vi "WSVCAP SHL Host LL I2C Write.vi"(0 "C1 Data Out [DUT Ordered]":u8[][](array[numeric]) format="%.0x", 1 "Wait Ticks":u32, 2 "Slave Address":u8, 5 "C2 Data Out [DUT Ordered]":u8[][](array[numeric]) format="%.0x", 7 "C3 Data Out [DUT Ordered]":u8[][](array[numeric]) format="%.0x", 9 "Socket Mask [U64]":u64=1 format="%016x", 11 "error in":errorcluster, 12 "Sub Address":u8=20, 13 "UUT Set (0/1)":u8) -> (10 "Status":u8[](array[numeric]), 15 "error out":errorcluster)   [LabVIEW 2012]
uses:
  Type Defs/WSVCAP SHL Top Level Write Read State Enum.ctl
  Type Defs/WSVCAP SHL Transaction Enum.ctl
  Type Defs/WSVCAP SHL Top Level Control Enum.ctl
  Type Defs/WSVCAP SHL State.ctl
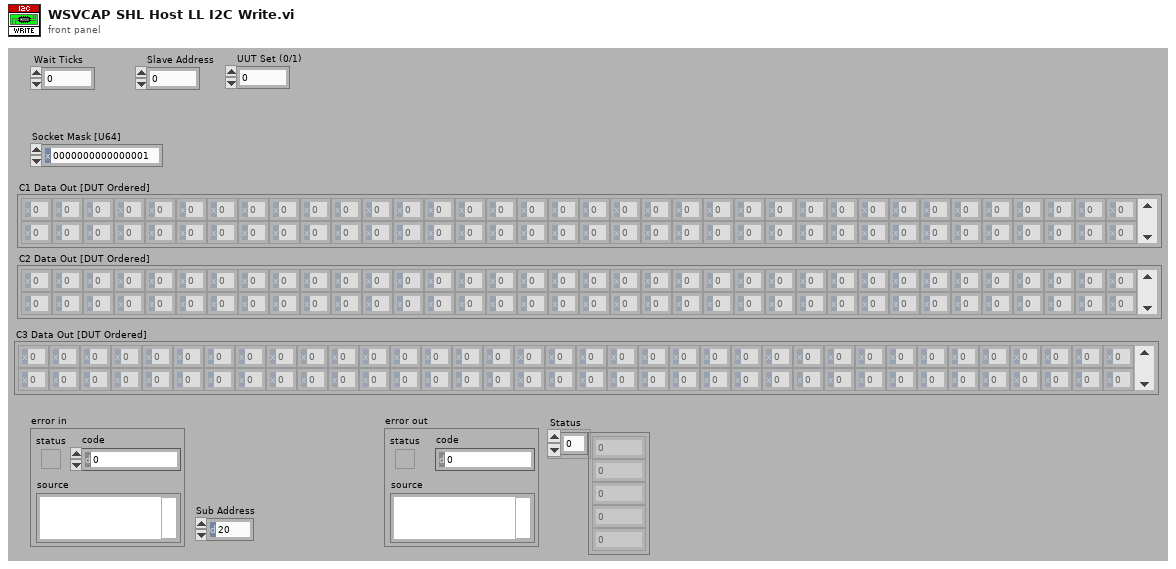
[diagram p1: front panel]
types:
  T1 = typedef "WSVCAP SHL Top Level Write Read State Enum.ctl" = enum16{"Start", "Write", "Read", "Get Status", "Wait Until Done"}
  T2 = typedef "WSVCAP SHL Top Level Control Enum.ctl" = enum16{"Start", "Cmd", "Transaction", "Wait Ticks", "Socket Mask", "UUT Set", "Slave Address", "Sub Address", "Bytes to Write", "Bytes to Read", "Write Data", "Write Flag", "Read Data", "Read Flag", "Ack Read", "Read Status Flag", "Ack Read Status", "Status", "Cycle Count", "Stop Cycle", "Exit"}
  T3 = typedef "WSVCAP SHL Transaction Enum.ctl" = enum16{"I2C-Read Data", "I2C-Write Data", "RFFE-Ext Write", "RFFE-Ext Read"}
  T4 = typedef "WSVCAP SHL State.ctl" = enum8{"Idle", "Transfer Data"}
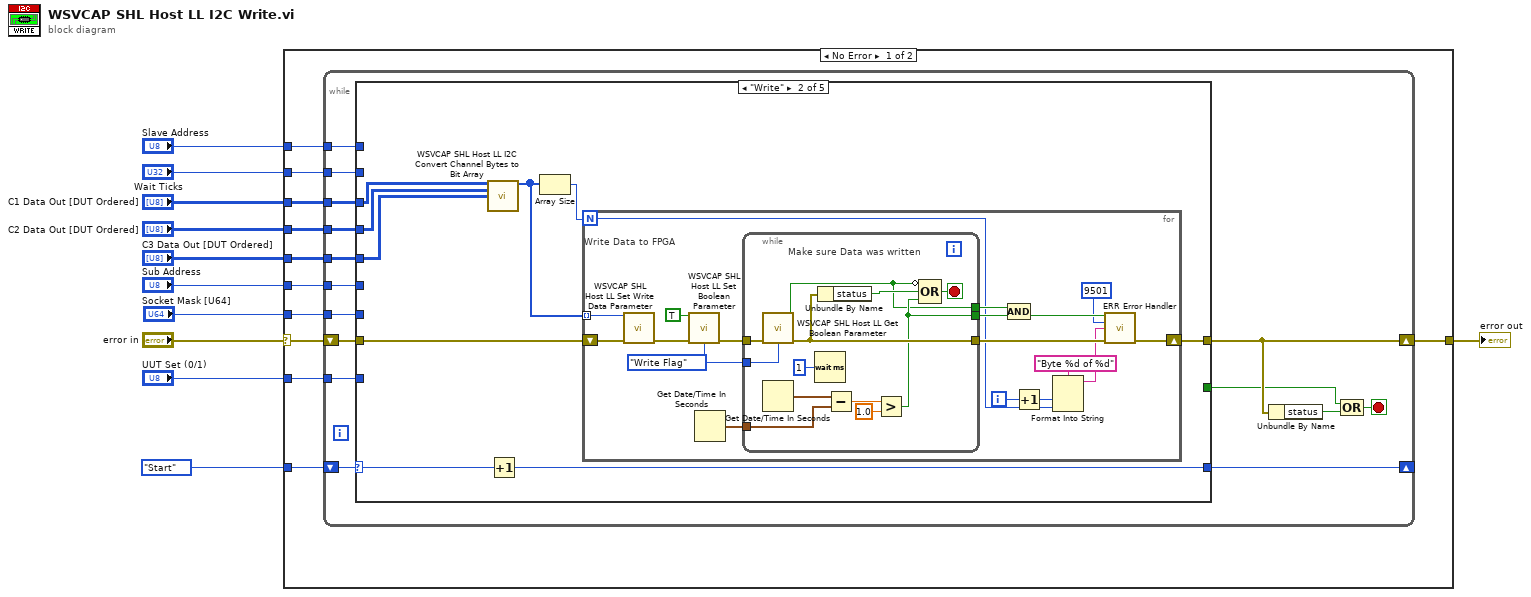
[diagram p0: block diagram]
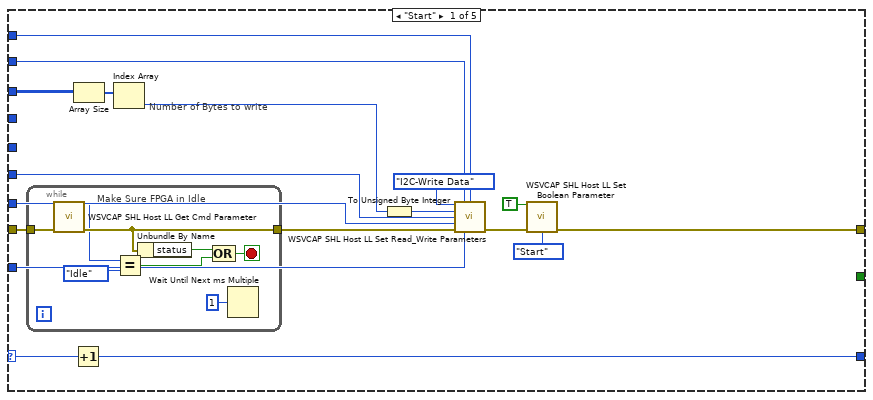
[diagram p2: hidden frame]
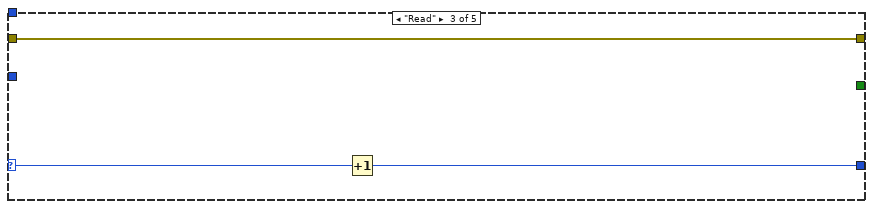
[diagram p3: hidden frame]
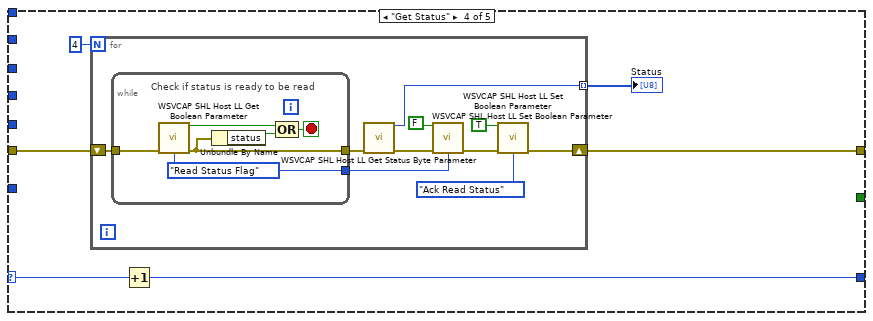
[diagram p4: hidden frame]
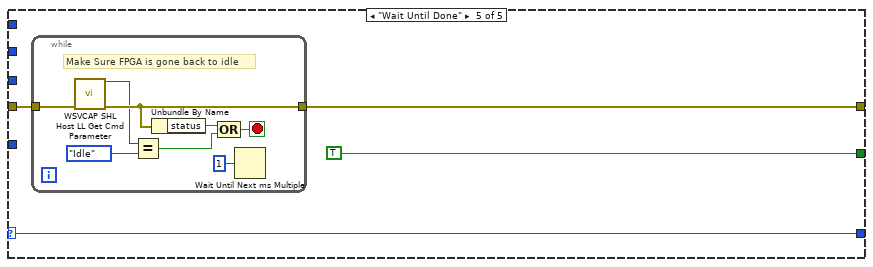
[diagram p5: hidden frame]
diagram:
  n1 = case shown="No Error" "error in" {
    selector: "error in" -> [w16 w139]
    tunnel: [w22 w139] -> w11
    tunnel: WSVCAP_SHL_Top_Level_Write_Read_State_Enum."Start" ("Write Read State") -> [w21 _]
    tunnel: "C1 Data Out [DUT Ordered]" -> [w20 _]
    tunnel: "C2 Data Out [DUT Ordered]" -> [w19 _]
    tunnel: "Sub Address" -> [w18 _]
    tunnel: "Socket Mask [U64]" -> [w17 _]
    tunnel: "Wait Ticks" -> [w15 _]
    tunnel: "C3 Data Out [DUT Ordered]" -> [w14 _]
    tunnel: "Slave Address" -> [w13 _]
    tunnel: "UUT Set (0/1)" -> [w12 _]
    frame No Error {
      n2 = while {
        shift-right: [w36] -> w22
        shift-left: w16 -> [w37]
        shift-right: [w31] -> _
        shift-left: w21 -> [w32]
        tunnel: w20 -> [w30]
        tunnel: w19 -> [w29]
        tunnel: w18 -> [w28]
        tunnel: w17 -> [w27]
        tunnel: w15 -> [w26]
        tunnel: w14 -> [w25]
        tunnel: w13 -> [w24]
        tunnel: w12 -> [w23]
        stop <- w33 stop-if-true
        n3 = case shown="\"Write\"" w32 {
          selector: w32 -> [w53 w69 w103 w108 w128]
          tunnel: w37 -> [w54 w66 w104 w110 w130]
          tunnel: [w50 w71 w104 w109 w129] -> w36
          tunnel: [_ _ _ _ TRUE] -> w35
          tunnel: [w52 w70 w102 w107 w128] -> w31
          tunnel: w30 -> [w46 w65 _ _ _]
          tunnel: w29 -> [_ w64 _ _ _]
          tunnel: w28 -> [w42 _ _ _ _]
          tunnel: w27 -> [w41 _ _ _ _]
          tunnel: w26 -> [w40 _ _ _ _]
          tunnel: w25 -> [_ w63 _ _ _]
          tunnel: w24 -> [w39 _ _ _ _]
          tunnel: w23 -> [w38 _ _ _ _]
          frame "Start" {
            # "Number of Bytes to write"
            n4 = while {
              tunnel: w54 -> [w58]
              tunnel: [w57] -> w51
              stop <- w62 stop-if-true
              # "Make Sure FPGA in Idle"
              n5 = call "WSVCAP SHL Host LL Get Cmd Parameter.vi"("error in (no error)"=w58) -> ("I2C_Cmd"=w56:T4, "error out"=w57:errorcluster)  [unwired: 13 in]
              n6 = Equal?(x=w56, y=WSVCAP_SHL_State."Idle" ("Type")) -> (x = y?=w60:bool)
              n7 = Unbundle By Name(w57) -> ("status"=w55:bool)
              n8 = Compound Arithmetic op=OR(w55, w60) -> (w62:bool)
              n9 = Wait Until Next ms Multiple(millisecond multiple=u32 1) -> ()  [unwired: 1 out]
            }
            n10 = Increment(x=w53) -> (x+1=w52:T1)
            n11 = Array Size(array=w46) -> (size(s)=w45:i32[])
            n12 = Index Array(array=w45) -> (element=w44:i32)  [unwired: 1 in]
            n13 = To Unsigned Byte Integer(number=w44) -> (unsigned 8bit integer=w43:u8)
            n14 = call "WSVCAP SHL Host LL Set Read_Write Parameters.vi"("Transaction"=WSVCAP_SHL_Transaction_Enum."I2C-Write Data", "Wait Ticks"=w40, "Slave Address"=w39, "Bytes"=w43, "Sub Address [U8]"=w42, "Socket Mask [U64]"=w41, "error in (no error)"=w51, "UUT Set (0/1)"=w38) -> ("error out"=w50:errorcluster)  [unwired: 7 in]
            n15 = call "WSVCAP SHL Host LL Set Boolean Parameter.vi"("Boolean In"=TRUE, "error in (no error)"=w50, "FPGA Top Level Control"=WSVCAP_SHL_Top_Level_Control_Enum."Start") -> ()  [unwired: 12 in, 1 out]
          }
          frame "Write" {
            # "Write Data to FPGA"
            n16 = call "WSVCAP SHL Host LL I2C Convert Channel Bytes to Bit Array.vi"("C1 Data Out"=w65, "C2 Data Out"=w64, "C3 Data Out"=w63) -> ("Write Data"=w67:u64[])  [unwired: 12 in]
            n17 = Increment(x=w69) -> (x+1=w70:T1)
            n18 = Array Size(array=w67) -> (size(s)=w68:i32)
            n19 = for {
              N: w68 -> [w73]
              shift-right: [w81] -> w71
              shift-left: w66 -> [w89]
              tunnel: w67 -> [w88] mode=indexing
              i -> [w76]
              w84 = WSVCAP_SHL_Top_Level_Control_Enum."Write Flag" ("FPGA Top Level Control")
              n20 = call "WSVCAP SHL Host LL Set Write Data Parameter.vi"("Write Byte In"=w88, "error in (no error)"=w89) -> ("error out"=w87:errorcluster)  [unwired: 13 in]
              n21 = call "WSVCAP SHL Host LL Set Boolean Parameter.vi"("Boolean In"=TRUE, "error in (no error)"=w87, "FPGA Top Level Control"=w84) -> ("error out"=w85:errorcluster)  [unwired: 12 in]
              n22 = Get Date/Time In Seconds() -> (seconds since 1Jan1904=w83:timestamp)
              n23 = while {
                tunnel: w85 -> [w99]
                tunnel: [w98] -> w82
                tunnel: w84 -> [w97]
                tunnel: w83 -> [w94]
                tunnel: [w91] -> w80
                tunnel: [w90] -> w79
                stop <- w101 stop-if-true
                # "Make sure Data was written"
                n24 = call "WSVCAP SHL Host LL Get Boolean Parameter.vi"("error in (no error)"=w99, "FPGA Top Level Control"=w97) -> ("Boolean Out"=w90:bool, "error out"=w98:errorcluster)  [unwired: 12 in]
                n25 = Get Date/Time In Seconds() -> (seconds since 1Jan1904=w95:timestamp)
                n26 = Wait (ms)(milliseconds to wait=u32 1) -> ()  [unwired: 1 out]
                n27 = Unbundle By Name(w98) -> ("status"=w96:bool)
                n28 = Subtract(x=w95, y=w94) -> (x-y=w93:dbl)
                n29 = Greater?(x=w93, y=1.0) -> (0:w91:bool)
                n30 = Compound Arithmetic op=OR(invert w90, w96, w91) -> (w101:bool)
              }
              n31 = Compound Arithmetic op=AND(w79, w80) -> (w78:bool)
              n32 = Increment(x=w76) -> (x+1=w72:i32)
              n33 = Format Into String(format string="Byte %d of %d", w72, w73) -> (resulting string=w75:string)  [unwired: 2 in, 1 out]
              n34 = call "ERR Error Handler.vi"("Error Status"=w78, "Error Code"=9501, "Cause Of Error"=w75, "Error In (no error)"=w82) -> ("Error Out"=w81:errorcluster)  [unwired: 11 in]
            }
          }
          frame "Read" {
            n35 = Increment(x=w103) -> (x+1=w102:T1)
          }
          frame "Get Status" {
            n36 = for {
              N: 4 -> [_]
              shift-right: [w119] -> w109
              shift-left: w110 -> [w120]
              tunnel: [w111] -> w105 mode=indexing
              n37 = while {
                tunnel: w120 -> [w124]
                tunnel: [w123] -> w118
                tunnel: [w121] -> w116
                stop <- w126 stop-if-true
                w121 = WSVCAP_SHL_Top_Level_Control_Enum."Read Status Flag" ("FPGA Top Level Control")
                # "Check if status is ready to be read"
                n38 = call "WSVCAP SHL Host LL Get Boolean Parameter.vi"("error in (no error)"=w124, "FPGA Top Level Control"=w121) -> ("Boolean Out"=w125:bool, "error out"=w123:errorcluster)  [unwired: 12 in]
                n39 = Unbundle By Name(w123) -> ("status"=w122:bool)
                n40 = Compound Arithmetic op=OR(w125, w122) -> (w126:bool)
              }
              n41 = call "WSVCAP SHL Host LL Get Status Byte Parameter.vi"("error in (no error)"=w118) -> ("I2C Status Byte"=w111:u8, "error out"=w117:errorcluster)  [unwired: 13 in]
              n42 = call "WSVCAP SHL Host LL Set Boolean Parameter.vi"("Boolean In"=FALSE ("Read Flag"), "error in (no error)"=w117, "FPGA Top Level Control"=w116) -> ("error out"=w112:errorcluster)  [unwired: 12 in]
              n43 = call "WSVCAP SHL Host LL Set Boolean Parameter.vi"("Boolean In"=TRUE ("Write Flag"), "error in (no error)"=w112, "FPGA Top Level Control"=WSVCAP_SHL_Top_Level_Control_Enum."Ack Read Status") -> ("error out"=w119:errorcluster)  [unwired: 12 in]
            }
            "Status" <- w105
            n44 = Increment(x=w108) -> (x+1=w107:T1)
          }
          frame "Wait Until Done" {
            n45 = while {
              tunnel: w130 -> [w133]
              tunnel: [w132] -> w129
              stop <- w135 stop-if-true
              # "Make Sure FPGA is gone back to idle"
              n46 = call "WSVCAP SHL Host LL Get Cmd Parameter.vi"("error in (no error)"=w133) -> ("I2C_Cmd"=w131:T4, "error out"=w132:errorcluster)  [unwired: 13 in]
              n47 = Equal?(x=w131, y=WSVCAP_SHL_State."Idle") -> (x = y?=w136:bool)
              n48 = Unbundle By Name(w132) -> ("status"=w137:bool)
              n49 = Compound Arithmetic op=OR(w137, w136) -> (w135:bool)
              n50 = Wait Until Next ms Multiple(millisecond multiple=u32 1) -> ()  [unwired: 1 out]
            }
          }
        }
        n51 = Unbundle By Name(w36) -> ("status"=w34:bool)
        n52 = Compound Arithmetic op=OR(w35, w34) -> (w33:bool)
      }
    }
    frame Error {
    }
  }
  "error out" <- w11
